vi "DSF.Engine.Runtime.Framework.Set Hardware Info.vi"(8 "error in (no error)":errorcluster, 10 "Hardware Info":refnum<class "DSF.Engine.Hardware Info.lvclass">, 11 "Framework Runtime in":refnum<class "DSF.Engine.Runtime.Framework.lvclass">) -> (0 "error out":errorcluster, 3 "Framework Runtime out":refnum<class "DSF.Engine.Runtime.Framework.lvclass">)   [LabVIEW 2016, in "DSF.Engine.lvlib" / "DSF.Engine.Runtime.Framework.lvclass"]
uses:
  DSF.Engine.Runtime.Framework.lvclass
  Hardware/DSF.Engine.Hardware Info.lvclass
  DSF.Engine.Runtime.Framework.lvclass/DSF.Engine.Runtime.Framework.ctl
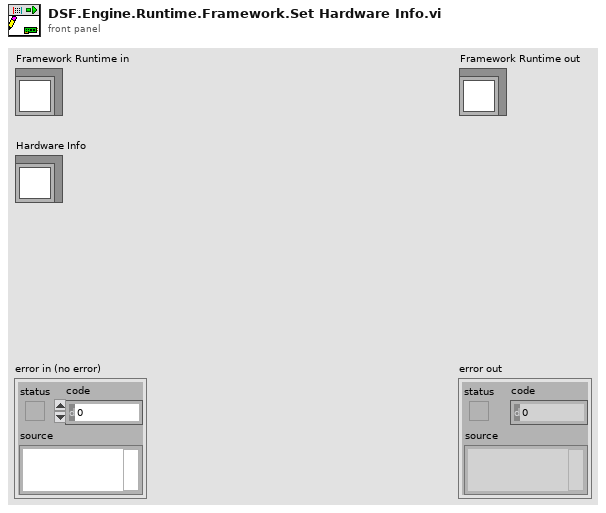
[diagram p1: front panel]
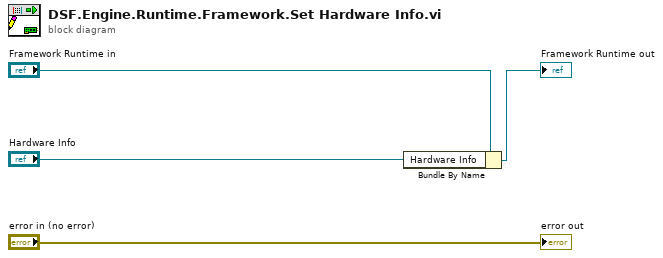
[diagram p0: block diagram]
diagram:
  n1 = Bundle By Name(cluster="Framework Runtime in", "Hardware Info"="Hardware Info") -> (→"Framework Runtime out":refnum<class "DSF.Engine.Runtime.Framework.lvclass">)
  "error out" <- "error in (no error)"
